vi "Refresh Display.vi"(6 "Local Data":T2 {"Acqusition Buffer"."Time Stamp" format="%<%x %.3X>T"}, 7 "QRD":T1, 8 "error in":errorcluster) -> (0 "error out":errorcluster, 4 "Local Data Out":T2 {"Acqusition Buffer"."Time Stamp" format="%<%x %.3X>T"}, 5 "QRD Out":T1)   [LabVIEW 2025]
uses:
  Controls/Local Data_Display.ctl
  Controls/Acquisition Packet.ctl
  Controls/Queues-Refs-Data.ctl
  Builds/Queue Wrappers.lvlibp/Q Packet.ctl
  Builds/Queue Wrappers.lvlibp
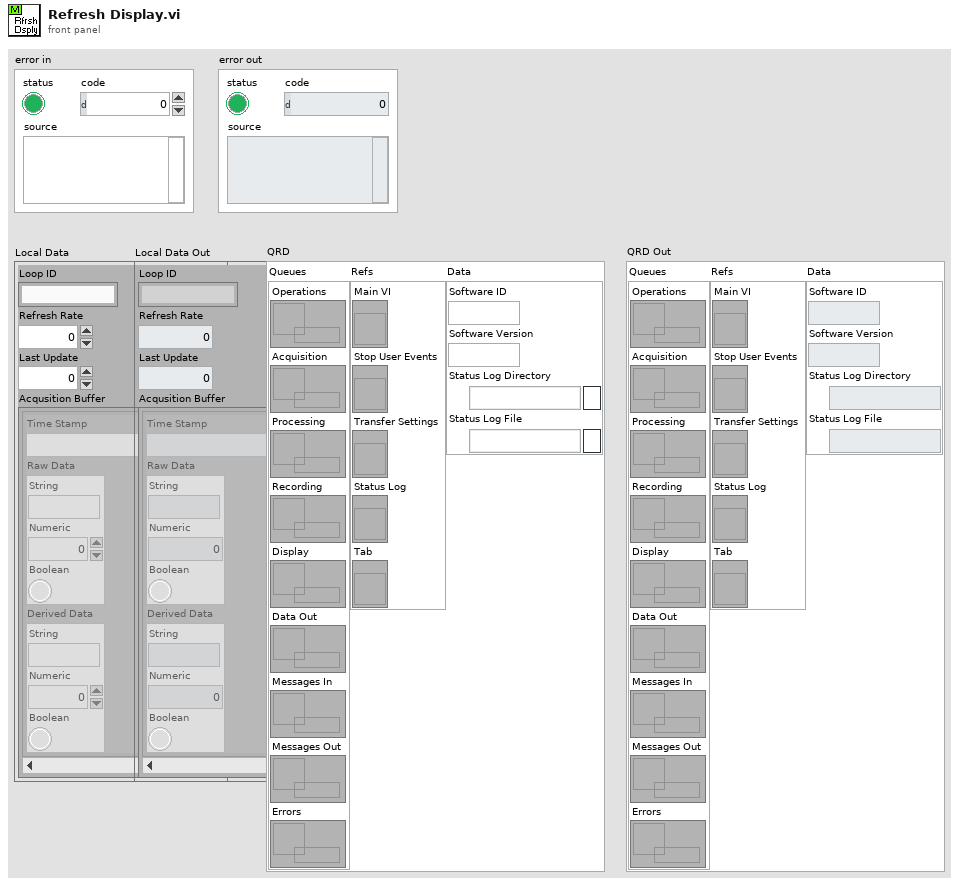
[diagram p1: front panel]
types:
  T1 = typedef "Queues-Refs-Data.ctl" = cluster{"Queues":cluster{"Operations":refnum<queue>, "Acquisition":refnum<queue>, "Processing":refnum<queue>, "Recording":refnum<queue>, "Display":refnum<queue>, "Data Out":refnum<queue>, "Messages In":refnum<queue>, "Messages Out":refnum<queue>, "Errors":refnum<queue>}, "Refs":cluster{"Main VI":refnum<vi>, "Stop User Events":refnum<vi>, "Transfer Settings":refnum<vi>, "Status Log":refnum<vi>, "Tab":refnum<vi>}, "Data":cluster{"Software ID":string, "Software Version":string, "Status Log Directory":path, "Status Log File":path}}
  T2 = typedef "Local Data_Display.ctl" = cluster{"Loop ID":string, "Refresh Rate":dbl, "Last Update":dbl, "Acqusition Buffer":T3[]}
  T3 = typedef "Acquisition Packet.ctl" = cluster{"Time Stamp":timestamp, "Raw Data":cluster{"String":string, "Numeric":dbl, "Boolean":bool}, "Derived Data":cluster{"String":string, "Numeric":dbl, "Boolean":bool}}
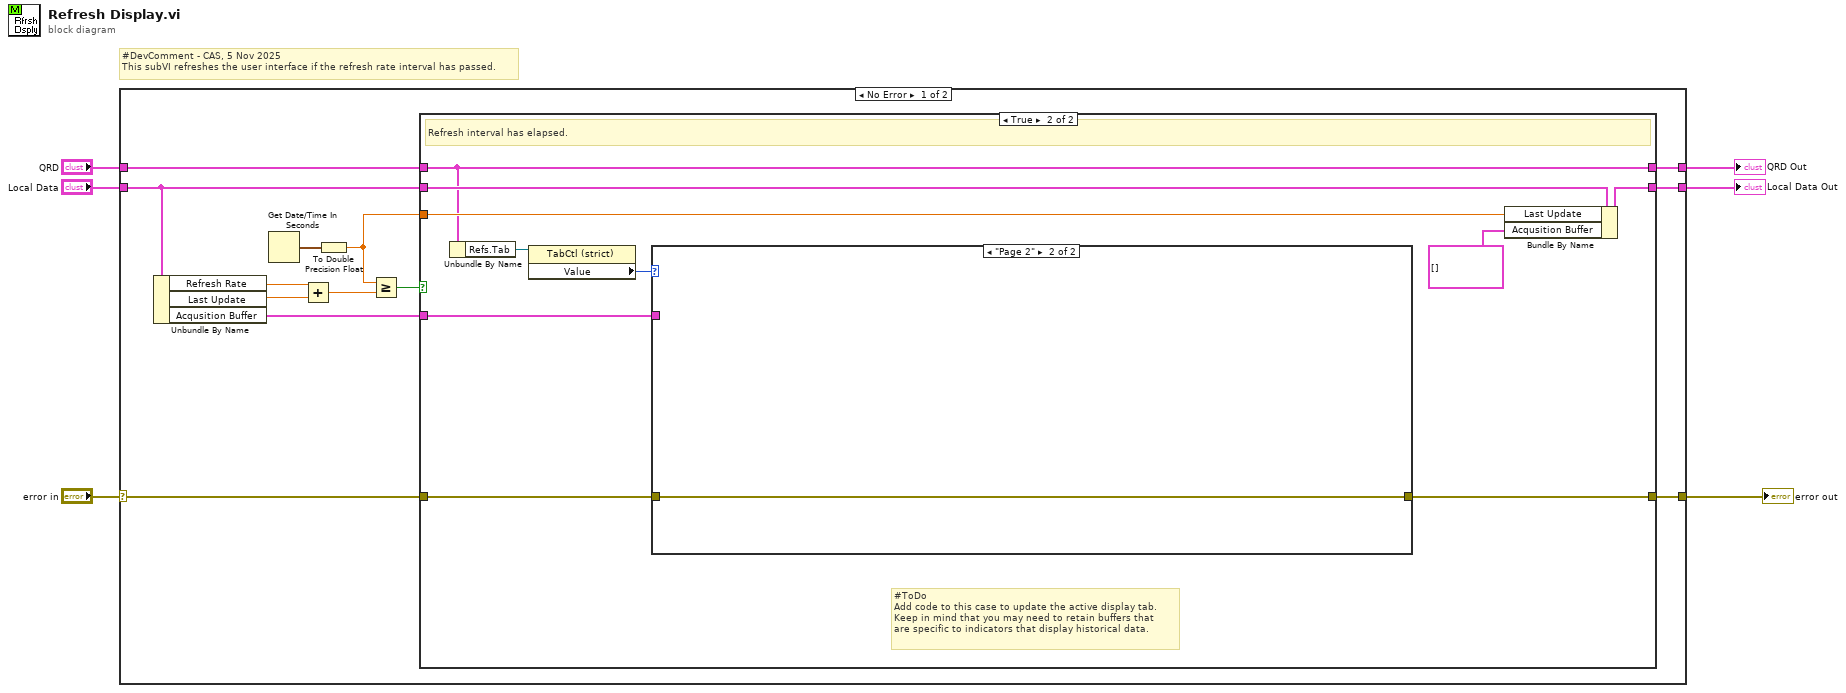
[diagram p0: block diagram]
diagram:
  # "#DevComment - CAS, 5 Nov 2025\nThis subVI refreshes the user interface if the refresh rate interval has passed."
  n1 = case shown="No Error" "error in" {
    selector: "error in" -> [w8 w35]
    tunnel: "Local Data" -> [w13 w37]
    tunnel: [w11 w37] -> w5
    tunnel: "QRD" -> [w10 w36]
    tunnel: [w9 w36] -> w3
    tunnel: [w7 w35] -> w1
    frame No Error {
      n2 = Unbundle By Name(w13) -> ("Refresh Rate"=w17:dbl, "Last Update"=w18:dbl, "Acqusition Buffer"=w12:T3[])
      n3 = Get Date/Time In Seconds() -> (seconds since 1Jan1904=w19:timestamp)
      n4 = Add(x=w17, y=w18) -> (x+y=w16:dbl)
      n5 = To Double Precision Float(number=w19) -> (double precision float=w14:dbl)
      n6 = Greater Or Equal?(x=w14, y=w16) -> (x >= y?=w15:bool)
      n7 = case shown="True" w15 {
        tunnel: w14 -> [_ w31]
        tunnel: w13 -> [w22 w32]
        tunnel: w12 -> [_ w25]
        tunnel: [w22 w29] -> w11
        tunnel: w10 -> [w21 w28]
        tunnel: [w21 w28] -> w9
        tunnel: w8 -> [w20 w24]
        tunnel: [w20 w23] -> w7
        frame False {
          # "Refresh interval has NOT elapsed."
        }
        frame True {
          # "#ToDo\nAdd code to this case to update the active display tab.\nKeep in mind that you may need to retain buffers that\nare specific to indicators that display historical data."
          # "Refresh interval has elapsed."
          n8 = Unbundle By Name(w28) -> ("Refs.Tab"=w27:refnum<vi>)
          n9 = property class="TabCtl (strict)"(reference=w27) -> ("Value"=w26:enum32{"Page 1", "Page 2", "Status Log"})  [unwired: 1 in, 2 out]
          n10 = case shown="\"Page 2\"" w26 {
            tunnel: w25 -> [_ _]
            tunnel: w24 -> [w33 w34]
            tunnel: [w33 w34] -> w23
            frame "Page 1", Default {
            }
            frame "Page 2" {
            }
          }
          n11 = Bundle By Name(cluster=w32, "Last Update"=w31, "Acqusition Buffer"=T3[] []) -> (w29:T2)
        }
      }
    }
    frame Error {
    }
  }
  "error out" <- w1
  "Local Data Out" <- w5
  "QRD Out" <- w3
